vi "HMI_GetTestInfoDialog.vi"(11 "RegTestInfo IN":T1) -> (3 "RegTestInfo Out":T1)   [LabVIEW 2024]
uses:
  Control Definitions/DEF_RegTestInfo.ctl
  Control Definitions/DEF_ConfigRings.ctl
panel:
  in  "Notes":string
  in  "Technician":string
  in  "Serial Number":string
  in  "Unit Number":string
  in  "Job Number":string
  out "Path":path[](array[path])
  in  "Test Report":u16(ring) items=["ReportTemplate_03.xltx", "***Search***"]
  in  "Test Configuration":u16(ring) items=["8005571-05 Elevate OLS .csv", "Level Rig ATP OLS-001 Config1.csv", "Level Rig ATP OLS-001 Config2.csv", "***Search***"]
  in  "Cancel":bool
  in  "OK":bool
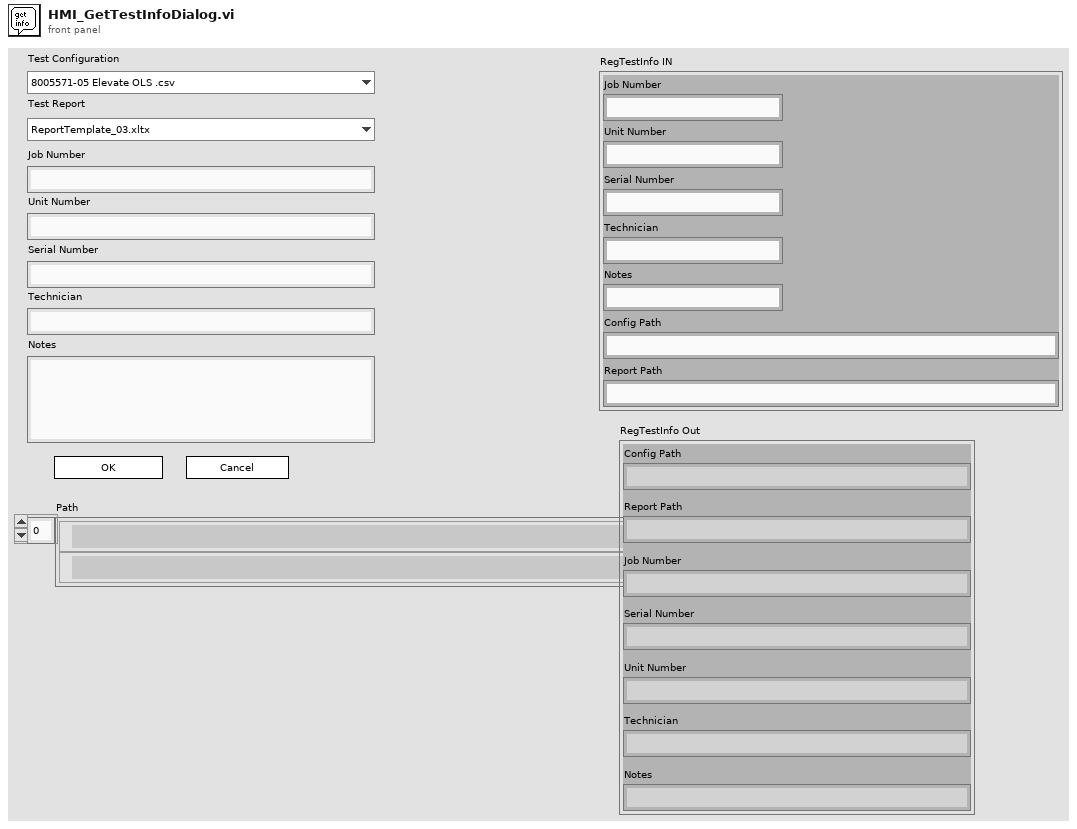
[diagram p1: front panel]
types:
  T1 = typedef "DEF_RegTestInfo.ctl" = cluster{"Job Number":string, "Unit Number":string, "Serial Number":string, "Technician":string, "Notes":string, "Config Path":string, "Report Path":string}
  T2 = typedef "DEF_ConfigRings.ctl" = cluster{"Ring Ctl":refnum<vi>, "Path":path, "Title":string, "Pattern":string, "Type":string}
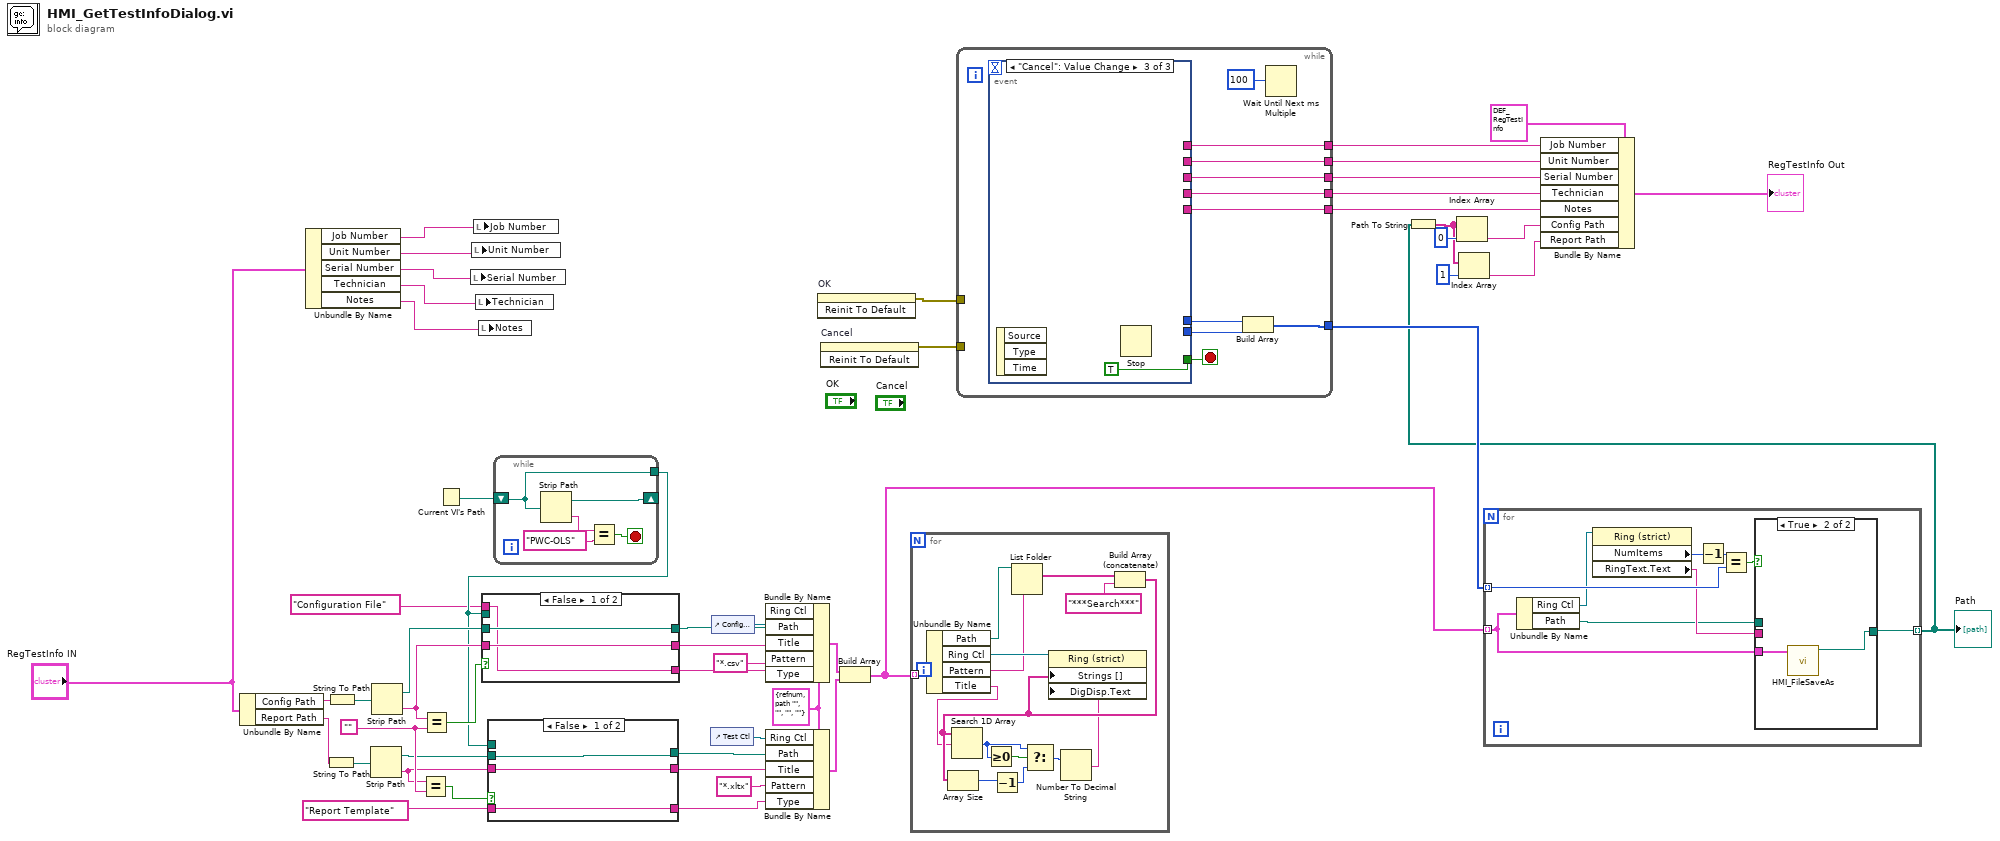
[diagram p0: block diagram]
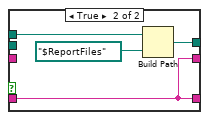
[diagram p2: hidden frame]
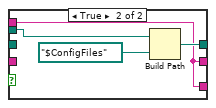
[diagram p3: hidden frame]
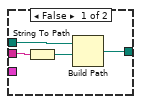
[diagram p4: hidden frame]
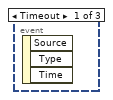
[diagram p5: hidden frame]
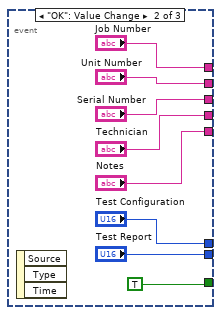
[diagram p6: hidden frame]
diagram:
  w34 = ""
  w45 = T2 {"Ring Ctl"=refnum, "Path"=path "", "Title"="", "Pattern"="", "Type"=""} ("output cluster")
  n1 = Unbundle By Name("RegTestInfo IN") -> ("Config Path"=w42:string, "Report Path"=w37:string)
  n2 = Unbundle By Name("RegTestInfo IN") -> ("Job Number"=w24:string, "Unit Number"=w23:string, "Serial Number"=w22:string, "Technician"=w21:string, "Notes"=w20:string)
  n3 = String To Path(string=w37) -> (path=w38:path)
  n4 = String To Path(string=w42) -> (path=w41:path)
  n5 = Strip Path(path=w38) -> (stripped path=w31:path, name=w30:string)
  n6 = Strip Path(path=w41) -> (stripped path=w28:path, name=w29:string)
  n7 = Equal?(x=w30, y=w34) -> (x = y?=w32:bool)
  n8 = Equal?(x=w29, y=w34) -> (x = y?=w33:bool)
  n9 = Current VI's Path() -> (path=w49:path)
  n10 = local write "Serial Number"(w22) -> ()
  n11 = local write "Unit Number"(w23) -> ()
  n12 = local write "Job Number"(w24) -> ()
  n13 = local write "Technician"(w21) -> ()
  n14 = local write "Notes"(w20) -> ()
  n15 = while {
    shift-right: [w56] -> _
    shift-left: w49 -> [w53]
    tunnel: [w53] -> w26
    stop <- w55 stop-if-true
    n16 = Strip Path(path=w53) -> (stripped path=w56:path, name=w52:string)
    n17 = Equal?(x=w52, y="PWC-OLS" ("String")) -> (x = y?=w55:bool)
  }
  n18 = case shown="False" w33 {
    tunnel: [w59 w60] -> w5
    tunnel: [w58 w63] -> w40
    tunnel: w26 -> [_ w61]
    tunnel: w29 -> [w59 _]
    tunnel: w28 -> [w58 _]
    tunnel: "Configuration File" ("Title") -> [w57 w60]
    tunnel: [w57 w60] -> w6
    frame False {
    }
    frame True {
      n19 = Build Path(base path=w61, name or relative path=path "$ConfigFiles" ("Path")) -> (appended path=w63:path)
    }
  }
  n20 = case shown="False" w32 {
    tunnel: [w65 w67] -> w3
    tunnel: w26 -> [_ w69]
    tunnel: [w66 w68] -> w39
    tunnel: w31 -> [w66 _]
    tunnel: w30 -> [w65 _]
    tunnel: "Report Template" ("Title") -> [w64 w67]
    tunnel: [w64 w67] -> w2
    frame False {
    }
    frame True {
      n21 = Build Path(base path=w69, name or relative path=path "$ReportFiles") -> (appended path=w68:path)
    }
  }
  n22 = control-ref of="Test Ctl"() -> (w47:refnum<vi>)
  n23 = control-ref of="Config Ctl"() -> (w44:refnum<vi>)
  n24 = Bundle By Name(cluster=w45, "Ring Ctl"=w44, "Path"=w40, "Title"=w5, "Pattern"="*.csv", "Type"=w6) -> (w46:T2)
  n25 = Bundle By Name(cluster=w45, "Ring Ctl"=w47, "Path"=w39, "Title"=w3, "Pattern"="*.xltx", "Type"=w2) -> (w48:T2)
  n26 = invoke on="OK" class="Bool" method="Reinit To Default"() -> (error out=w51:errorcluster)  [unwired: 3 in, 2 out]
  n27 = invoke on="Cancel" class="Bool" method="Reinit To Default"() -> (error out=w50:errorcluster)  [unwired: 3 in, 2 out]
  n28 = Build Array(w46, w48) -> (w1:T2[])
  n29 = for {
    tunnel: w1 -> [w82] mode=indexing
    n30 = Unbundle By Name(w82) -> ("Path"=w80:path, "Ring Ctl"=w81:refnum<vi>, "Pattern"=w71:string, "Title"=w72:string)
    n31 = List Folder(path=w80, pattern=w71) -> (filenames=w84:string[])  [unwired: 2 in, 3 out]
    n32 = Build Array (concatenate)(w84, "***Search***") -> (w74:string[])
    n33 = Array Size(array=w74) -> (size(s)=w76:i32)
    n34 = Search 1D Array(1D array=w74, element=w72) -> (index of element=w78:i32)  [unwired: 1 in]
    n35 = Greater Or Equal To 0?(x=w78) -> (x >= 0?=w79:bool)
    n36 = Decrement(x=w76) -> (x-1=w75:i32)
    n37 = Select(t=w78, s=w79, f=w75) -> (s? t:f=w77:i32)
    n38 = Number To Decimal String(number=w77) -> (decimal integer string=w73:string)  [unwired: 1 in]
    n39 = property class="Ring (strict)"(reference=w81, "Strings []"=w74, "DigDisp.Text"=w73) -> ()  [unwired: 1 in, 2 out]
  }
  n40 = while {
    tunnel: w51 -> [_]
    tunnel: w50 -> [_]
    tunnel: [w93] -> w43
    tunnel: [w87] -> w13
    tunnel: [w88] -> w12
    tunnel: [w89] -> w11
    tunnel: [w90] -> w10
    tunnel: [w91] -> w9
    stop <- w92 stop-if-true
    n41 = event shown="[2] \"Cancel\": Value Change" {
      selector: _ -> [_ _ _]
      dyn-events: _ -> [_ _ _]
      timeout: _ -> [_ _ _]
      tunnel: [_ TRUE TRUE] -> w92
      tunnel: [_ "Notes" _] -> w91
      tunnel: [_ "Technician" _] -> w90
      tunnel: [_ "Serial Number" _] -> w89
      tunnel: [_ "Unit Number" _] -> w88
      tunnel: [_ "Job Number" _] -> w87
      tunnel: [_ "Test Report" _] -> w86
      tunnel: [_ "Test Configuration" _] -> w85
      event Timeout {
        n42 = event-data() -> ()  [unwired: 1 in, 3 out]
      }
      event "OK": Value Change {
        n43 = event-data() -> ()  [unwired: 1 in, 3 out]
      }
      event "Cancel": Value Change {
        n44 = event-data() -> ()  [unwired: 1 in, 3 out]
        n45 = Stop() -> ()  [unwired: 1 in]
      }
    }
    n46 = Build Array(w85, w86) -> (w93:u16[])
    n47 = Wait Until Next ms Multiple(millisecond multiple=100) -> ()  [unwired: 1 out]
  }
  n48 = for {
    tunnel: w43 -> [w110] mode=indexing
    tunnel: [w112] -> w27 mode=indexing
    tunnel: w1 -> [w104] mode=indexing
    n49 = Unbundle By Name(w104) -> ("Ring Ctl"=w106:refnum<vi>, "Path"=w105:path)
    n50 = property class="Ring (strict)"(reference=w106) -> ("NumItems"=w108:u32, "RingText.Text"=w107:string)  [unwired: 1 in, 2 out]
    n51 = Decrement(x=w108) -> (x-1=w109:u32)
    n52 = Equal?(x=w109, y=w110) -> (x = y?=w111:bool)
    n53 = case shown="True" w111 {
      tunnel: [w114 w117] -> w112
      tunnel: w105 -> [w115 _]
      tunnel: w107 -> [w113 _]
      tunnel: w104 -> [_ w118]
      frame False {
        n54 = String To Path(string=w113) -> (path=w116:path)
        n55 = Build Path(base path=w115, name or relative path=w116) -> (appended path=w114:path)
      }
      frame True {
        n56 = call "HMI_FileSaveAs.vi"("File Info"=w118) -> ("selected path"=w117:path)  [unwired: 10 in]
      }
    }
  }
  "Path" <- w27
  n57 = Path To String(path=w27) -> (string=w16:string[])
  n58 = Index Array(array=w16, index=0) -> (element=w15:string)
  n59 = Index Array(array=w16, index=1) -> (element=w14:string)
  n60 = Bundle By Name(cluster=T1 {"Job Number"="", "Unit Number"="", "Serial Number"="", "Technician"="", "Notes"="", "Config Path"="C:\\AllenProjects\\PWC-OLS\\$ConfigFiles\\8005571-05 Elevate OLS .csv", "Report Path"="C:\\AllenProjects\\PWC-OLS\\$ConfigFiles\\8005571-05 Elevate OLS .csv"} ("RegTestInfo IN"), "Job Number"=w13, "Unit Number"=w12, "Serial Number"=w11, "Technician"=w10, "Notes"=w9, "Config Path"=w15, "Report Path"=w14) -> (→"RegTestInfo Out":T1)
